vi "Load 3D tiff stack.vi"(1 "Image File":path=path "C:/My LabVIEW/Thumbnail Grid Hooovahh edit/Native Test/images/address-book-new.png") -> (0 "24-bit pixmap":u32[][][](array[numeric]))   [LabVIEW 2019]
doc: "This demo VI shows the functionality that the .NET PictureBox has when displaying images on a front panel. This VI can display any <B>Image File</B> into the PictureBox control, and then automatically control the <B>Size Mode (Zoom)</B> without any additional LabVIEW code. This demo VI also shows the opacity feature with <B>Grey Out Image?</B>, and the <B>Background Color</B>.\n\n-----\nBrian Hoover (hooovahh)"
uses:
  System.Windows.Forms
  System.Drawing
panel:
  in  "PictureBox":refnum<k24>(container)
  out "Number Of Images":i32
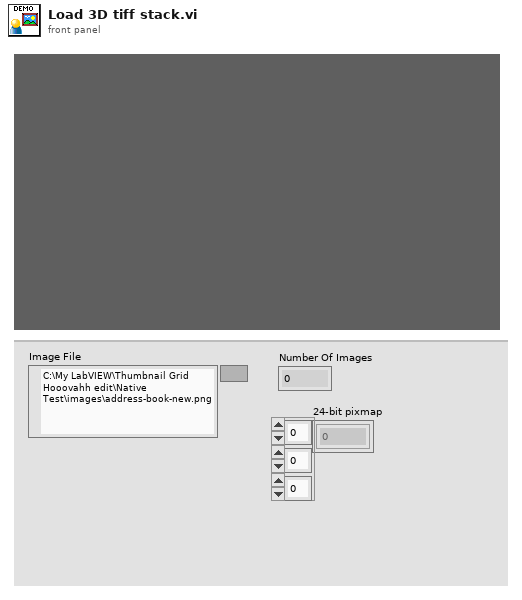
[diagram p1: front panel]
types:
  T1 = typedef "imagedata.ctl" = cluster{"image type":i32, "image depth":i32, "image":u8[], "mask":u8[], "colors":u32[], "Rectangle":cluster{"left":i16, "top":i16, "right":i16, "bottom":i16}}
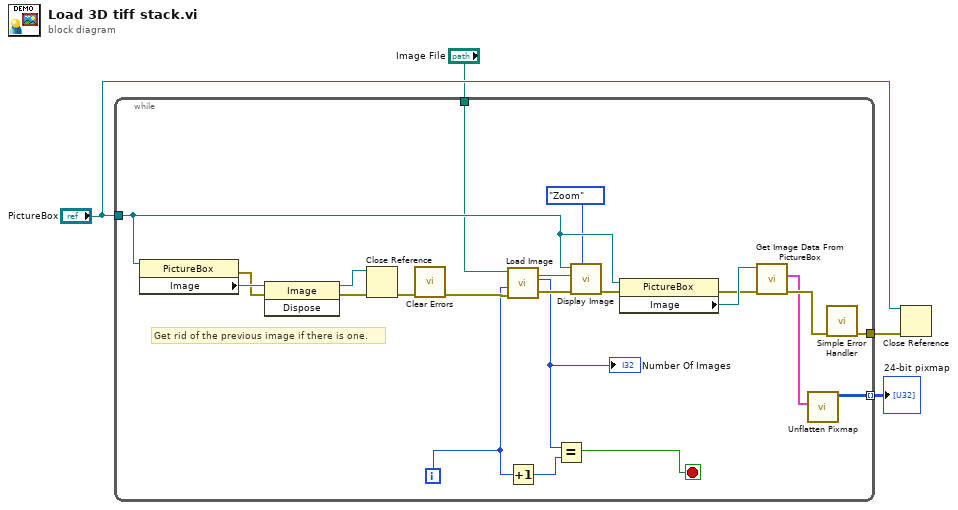
[diagram p0: block diagram]
diagram:
  n1 = while {
    tunnel: "PictureBox" -> [w26]
    tunnel: [w25] -> w3
    tunnel: "Image File" -> [w10]
    tunnel: [w5] -> w1 mode=indexing
    i -> [w9]
    stop <- w6 stop-if-true
    # "Get rid of the previous image if there is one."
    n2 = property class="PictureBox"(reference=w26) -> (error out=w14:errorcluster, "Image"=w18:refnum<k24>)  [unwired: 1 in, 1 out]
    n3 = invoke class="Image" method="Dispose"(reference=w18, error in=w14) -> (reference out=w15:refnum<k24>, error out=w16:errorcluster)  [unwired: 1 in, 1 out]
    n4 = Close Reference(reference=w15, error in (no error)=w16) -> (error out=w17:errorcluster)
    n5 = call <vilib>:"Clear Errors.vi"("error in (no error)"=w17) -> ("error out"=w11:errorcluster)  [unwired: 5 in, 1 out]
    n6 = call "Load Image.vi"("error in (no error)"=w11, "Image Index"=w9, "Image File"=w10) -> ("error out"=w23:errorcluster, "Number Of Images"=w8:i32, "Image"=w24:refnum<k24>)  [unwired: 6 in]
    "Number Of Images" <- w8
    n7 = Increment(x=w9) -> (x+1=w7:i32)
    n8 = Equal?(x=w8, y=w7) -> (x = y?=w6:bool)
    n9 = call "Display Image.vi"("Size Mode (Zoom)"=enum16{"Normal", "Stretch", "Center", "Zoom"}."Zoom", "error in (no error)"=w23, "Image"=w24, "PictureBox"=w26) -> ("error out"=w22:errorcluster)  [unwired: 6 in, 1 out]
    n10 = property class="PictureBox"(reference=w26, error in=w22) -> (error out=w20:errorcluster, "Image"=w21:refnum<k24>)  [unwired: 1 out]
    n11 = call "Get Image Data From PictureBox.vi"("error in (no error)"=w20, "Image"=w21) -> ("error out"=w19:errorcluster, "Image Data"=w12:T1)  [unwired: 7 in, 1 out]
    n12 = call <vilib>:"Unflatten Pixmap.vi"("image data"=w12) -> ("24-bit pixmap"=w5:u32[][])  [unwired: 4 in, 6 out]
    n13 = call <vilib>:"Simple Error Handler.vi"("error in (no error)"=w19) -> ("error out"=w25:errorcluster)  [unwired: 4 in, 4 out]
  }
  "24-bit pixmap" <- w1
  n14 = Close Reference(reference="PictureBox", error in (no error)=w3) -> ()  [unwired: 1 out]
